vi "State2016.vi"() -> ()   [LabVIEW 2017]
panel:
  out "emergency":bool
  out "gear":dbl
  out "y":dbl
  out "x":dbl
  out "y_dot":dbl
  out "x_dot":dbl
  out "yaw_rate":dbl
  out "heading":dbl
  out "angular_velocity":dbl
  out "lon_acc":dbl
  out "lat_acc":dbl
  out "turning_radius":dbl
  out "wheel_angle":dbl
  out "rear_right_wheel":dbl
  out "rear_left_wheel":dbl
  out "front_right_wheel":dbl
  out "front_left_wheel":dbl
  out "velocity":dbl
  # "state2016"
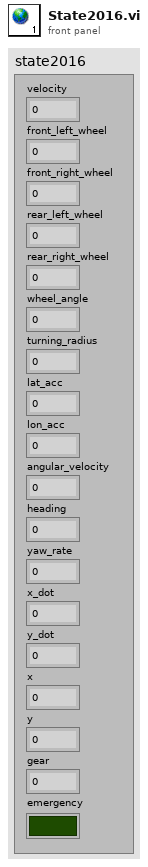
[diagram p1: front panel]
diagram:
